vi "Mes Select Cmd.vi"(0 "DateInfo":string, 1 "h/r":bool, 5 "Shift":string, 7 "Line_Name":string, 9 "AvaType":string, 11 "error in (no error)":errorcluster) -> (4 "resulting string":string, 15 "error out":errorcluster)   [LabVIEW 2014]
panel:
  # "and DateInfo='%1$s' and Shift='%2$s' \nand Line_Name ='%3$s'  and AvaType ='%4$s'"
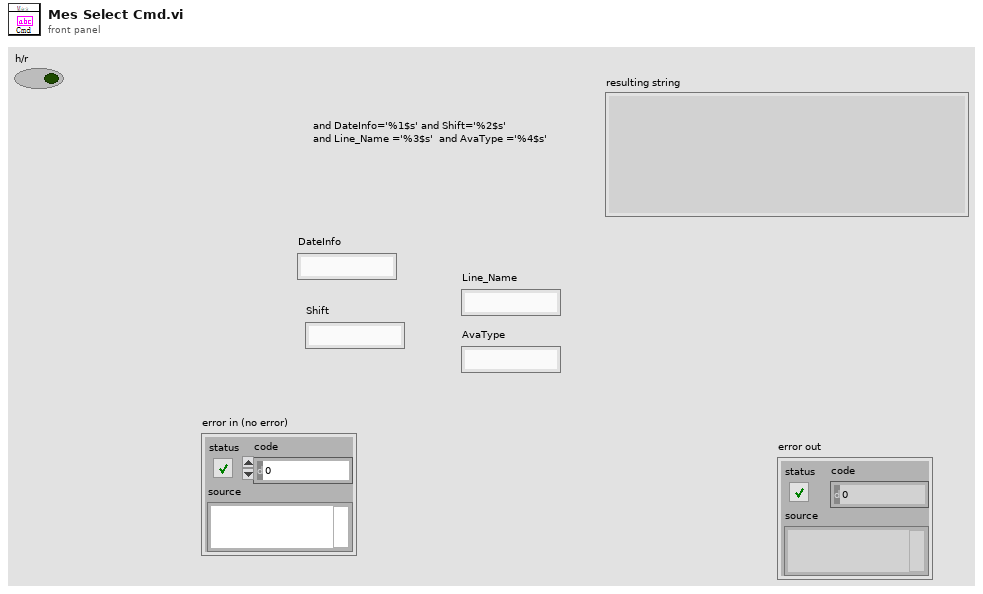
[diagram p1: front panel]
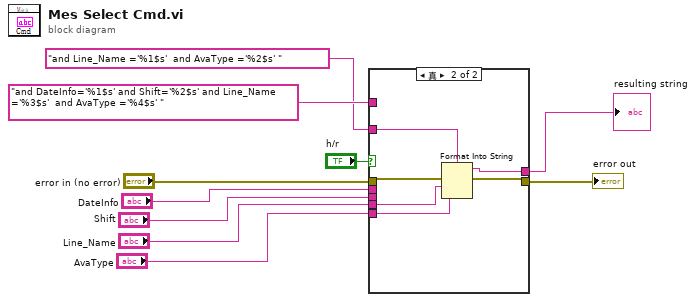
[diagram p0: block diagram]
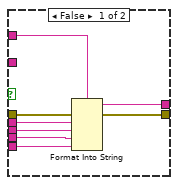
[diagram p2: hidden frame]
diagram:
  n1 = case shown="真" "h/r" {
    tunnel: "and DateInfo='%1$s' and Shift='%2$s' and Line_Name ='%3$s'  and AvaType ='%4$s' " -> [w18 _]
    tunnel: "error in (no error)" -> [w17 w24]
    tunnel: "DateInfo" -> [w16 _]
    tunnel: "Shift" -> [w15 _]
    tunnel: "Line_Name" -> [w14 w20]
    tunnel: "AvaType" -> [w13 w19]
    tunnel: [w12 w22] -> w4
    tunnel: [w11 w23] -> w3
    tunnel: "and Line_Name ='%1$s'  and AvaType ='%2$s' " -> [_ w21]
    frame False {
      n2 = Format Into String(format string=w18, error in=w17, w16, w15, w14, w13) -> (resulting string=w12:string, error out=w11:errorcluster)  [unwired: 1 in]
    }
    frame True {
      n3 = Format Into String(format string=w21, error in=w24, w20, w19) -> (resulting string=w22:string, error out=w23:errorcluster)  [unwired: 1 in]
    }
  }
  "error out" <- w3
  "resulting string" <- w4
